vi "SelectRectangularRegion.vi"() -> ()   [LabVIEW 2017]
uses:
  <vilib>/vision/NI_Vision_Development_Module.lvlib
panel:
  out "Blue Avg.":dbl
  out "Green Avg.":dbl
  out "Red Avg.":dbl
  out "Blue":u32[][](array[numeric])
  out "Green":u32[][](array[numeric])
  out "Red":u32[][](array[numeric])
  out "Y Resolution":i32
  out "X Resolution":i32
  out "Image Pixels (U32)":u32[][](array[numeric])
  out "Rectangular region":T1(plugin-control)
  out "error out":errorcluster
  out "Original Image":T1(plugin-control)
  in  "File Path":path
  in  "error in":errorcluster
  # "High byte is the alpha value"
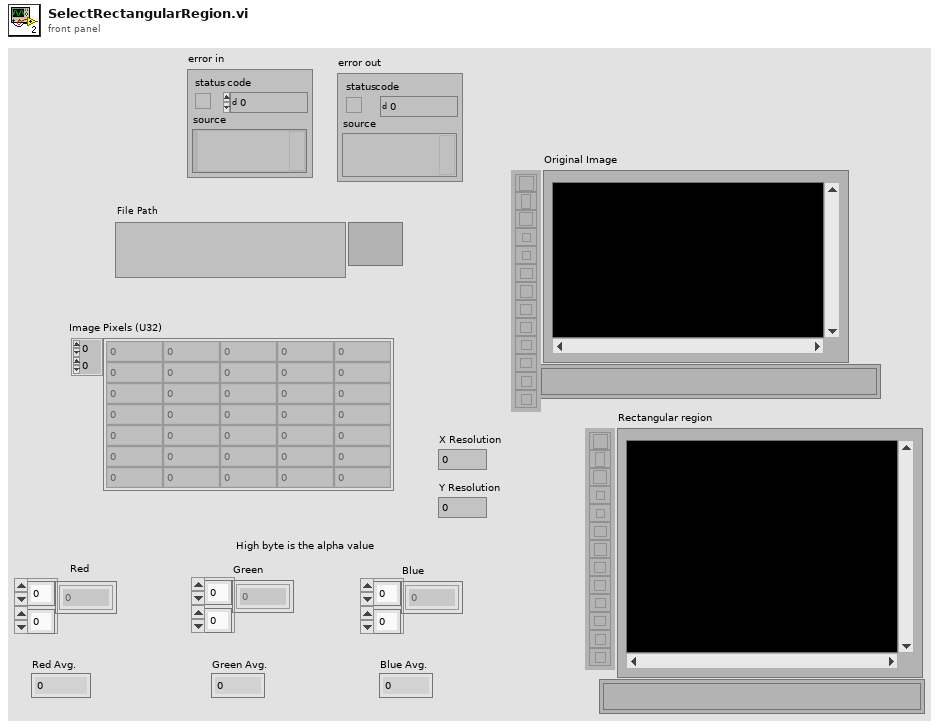
[diagram p1: front panel]
types:
  T1 = typedef "IMAQ Image.ctl" = refnum<image>
  T2 = typedef "Image Type" = u32
  T3 = typedef "IMAQ Rectangle" = cluster{"Left":i32, "Top":i32, "Right":i32, "Bottom":i32, "Rotation":dbl}
  T4 = typedef "ROI Descriptor" = cluster{"Global Rectangle":i32[], "Contours":cluster{"ID":enum32{"External", "Internal"}, "Type":u32, "Coordinates":i32[]}[]}
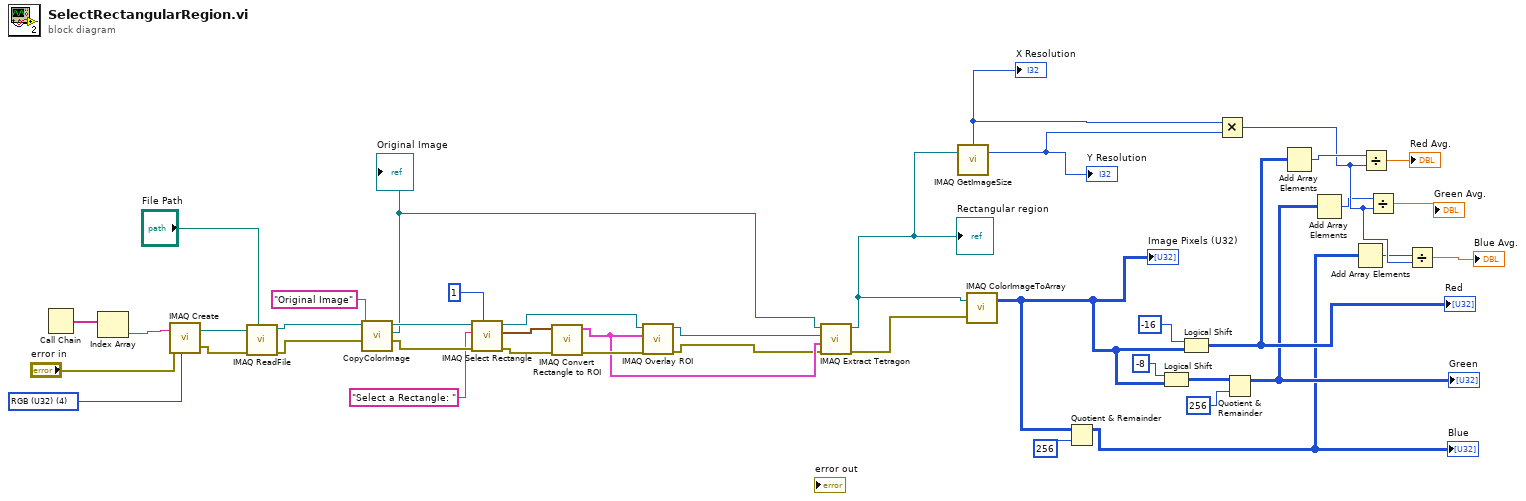
[diagram p0: block diagram]
diagram:
  w42 = T2 4 items=["Grayscale (U8)", "Grayscale (I16)", "Grayscale (SGL)", "Complex (CSG)", "RGB (U32)", "HSL (U32)", "RGB (U64)", "Grayscale (U16)"] ("Image Type")
  n1 = Call Chain() -> (call chain=w41:string[])
  n2 = Index Array(array=w41) -> (element=w40:string)  [unwired: 1 in]
  n3 = call "IMAQ Create"("Image Name"=w40, "Image Type"=w42, "error in (no error)"="error in") -> ("New Image"=w39:T1, "error out"=w38:errorcluster)  [unwired: 2 in]
  n4 = call "IMAQ ReadFile"("File Path"="File Path", "error in (no error)"=w38, "Image"=w39) -> ("error out"=w33:errorcluster, "Image Out"=w35:T1)  [unwired: 2 in, 5 out]
  n5 = call "CopyColorImage.vi"("Error in 1"=w33, "Image Name"="Original Image", "Image"=w35) -> ("error out 2"=w31:errorcluster, "Out 2"=w24:T1, "Out"=w32:T1)  [unwired: 5 in, 1 out]
  "Original Image" <- w24
  n6 = call "IMAQ Select Rectangle"("Window Number (0...15)"=1, "error in (no error)"=w31, "Prompt"="Select a Rectangle: ", "Image In"=w32) -> ("error out"=w27:errorcluster, "Rectangle"=w28:T3, "Image Out (duplicate)"=w25:T1)  [unwired: 4 in, 1 out]
  n7 = call "IMAQ Convert Rectangle to ROI"("error in (no error)"=w27, "Rectangle"=w28) -> ("error out"=w26:errorcluster, "ROI Descriptor"=w23:T4)  [unwired: 7 in]
  n8 = call "IMAQ Overlay ROI"("error in (no error)"=w26, "ROI Descriptor"=w23, "Image"=w25) -> ("error out"=w22:errorcluster, "Image Out"=w21:T1)  [unwired: 7 in]
  n9 = call-poly "IMAQ Extract Tetragon"("error in (no error)"=w22, "ROI Descriptor"=w23, "Image Dst"=w21, "Image Src"=w24) -> ("error out"=w20:errorcluster, "Image Dst Out"=w19:T1)  [unwired: 6 in]
  "Rectangular region" <- w19
  n10 = call "IMAQ GetImageSize"("Image"=w19) -> ("Y Resolution"=w11:i32, "X Resolution"=w12:i32)  [unwired: 3 in, 1 out]
  "X Resolution" <- w12
  "Y Resolution" <- w11
  n11 = call "IMAQ ColorImageToArray"("Image"=w19, "error in (no error)"=w20) -> ("Image Pixels (U32)"=w14:u32[][])  [unwired: 2 in, 2 out]
  "Image Pixels (U32)" <- w14
  n12 = Quotient & Remainder(x=w14, y=u32 256) -> (x-y*floor(x/y)=w5:u32[][])  [unwired: 1 out]
  "Blue" <- w5
  n13 = Logical Shift(y=i16 -8, x=w14) -> (x << y=w15:u32[][])
  n14 = Logical Shift(y=i16 -16, x=w14) -> (x << y=w10:u32[][])
  "Red" <- w10
  n15 = Multiply(x=w12, y=w11) -> (x*y=w7:i32)
  n16 = Quotient & Remainder(x=w15, y=u32 256) -> (x-y*floor(x/y)=w6:u32[][])  [unwired: 1 out]
  "Green" <- w6
  n17 = Add Array Elements(numeric array=w10) -> (sum=w9:u32)
  n18 = Add Array Elements(numeric array=w6) -> (sum=w4:u32)
  n19 = Add Array Elements(numeric array=w5) -> (sum=w3:u32)
  n20 = Divide(x=w9, y=w7) -> (x/y=→"Red Avg.":dbl)
  n21 = Divide(x=w4, y=w7) -> (x/y=→"Green Avg.":dbl)
  n22 = Divide(x=w3, y=w7) -> (x/y=→"Blue Avg.":dbl)
